vi "Facade.vi"(0 "Data In":T4, 2 "Display State In":T2, 3 "Container State":T3) -> (6 "Data Out":T4, 7 "Display State Out":T2, 8 "Action":T1)   [LabVIEW 2015, in "SAM.xctl"]
uses:
  SAM.xctl
  Data.vi
  Classes/Modulations/SAM/SAM.lvclass
  <vilib>/_xctls/Container State.ctl
  State.vi
  <vilib>/_xctls/Action.ctl
  Classes/Modulations/SAM/SAM.lvclass/SAM.ctl
  Classes/Modulations/SAM/Read Frequency (Hz).vi
  Classes/Modulations/SAM/Read Phase (0-1).vi
  Classes/Modulations/SAM/Write Frequency (Hz).vi
  Classes/Modulations/SAM/Write Phase (0-1).vi
  <vilib>/_xctls/XControlSupport.lvlib
panel:
  in  "Phase (cycles)":dbl min=0.0 max=1.0
  in  "Frequency (Hz)":dbl
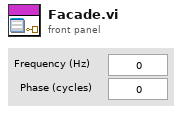
[diagram p1: front panel]
types:
  T1 = typedef "XControlSupport.lvlib/Action.ctl" = cluster{"Data Changed?":bool, "State Changed?":bool, "Action Name":string}
  T2 = typedef "SAM.xctl/State.vi" = cluster{"Numeric":dbl}
  T3 = typedef "XControlSupport.lvlib/Container State.ctl" = cluster{"Indicator?":bool, "Run Mode?":bool, " Refnum":refnum<vi>}
  T4 = typedef "SAM.xctl/Data.vi" = refnum<class "SAM.lvclass">
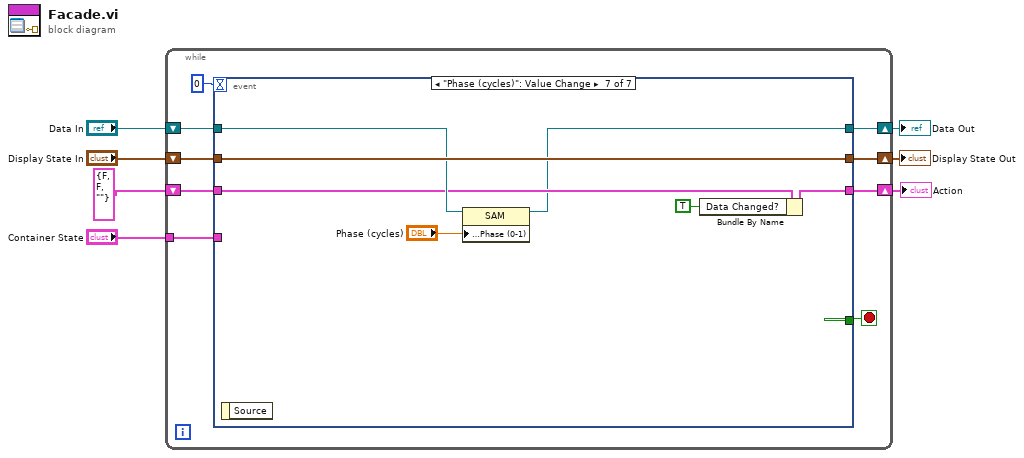
[diagram p0: block diagram]
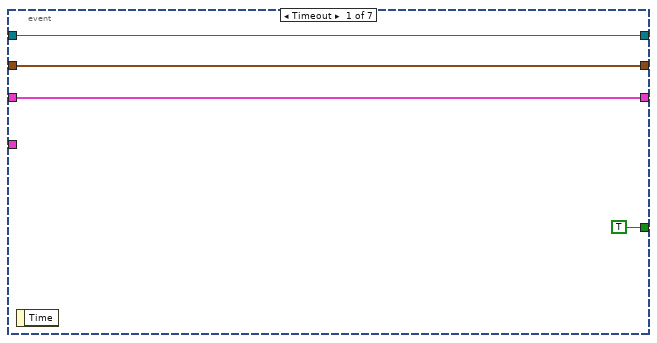
[diagram p2: hidden frame]
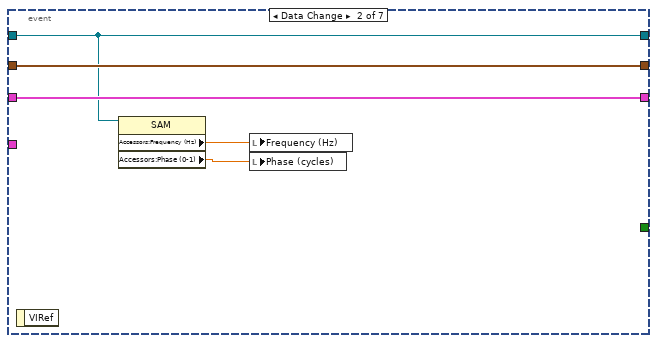
[diagram p3: hidden frame]
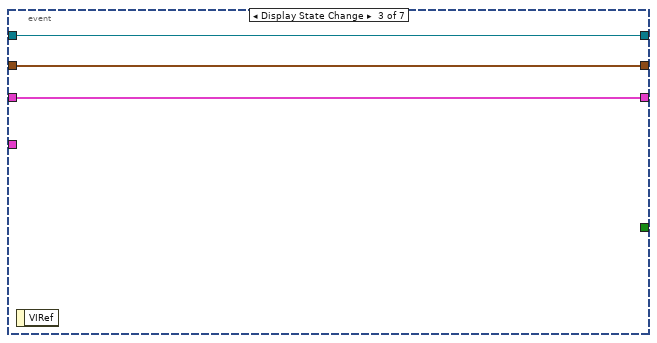
[diagram p4: hidden frame]
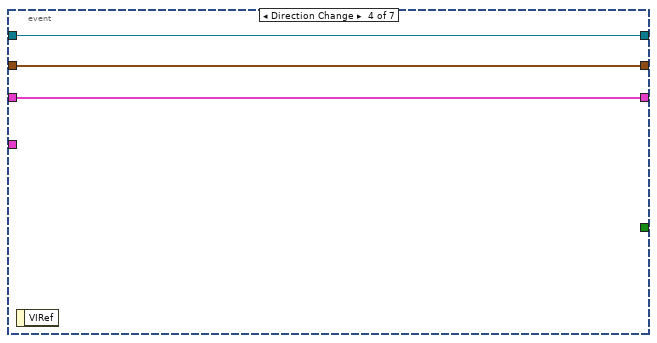
[diagram p5: hidden frame]
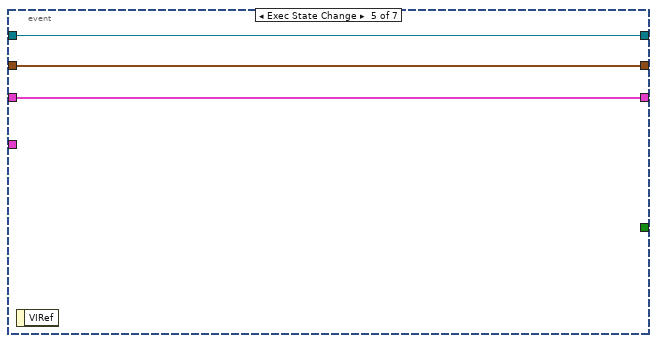
[diagram p6: hidden frame]
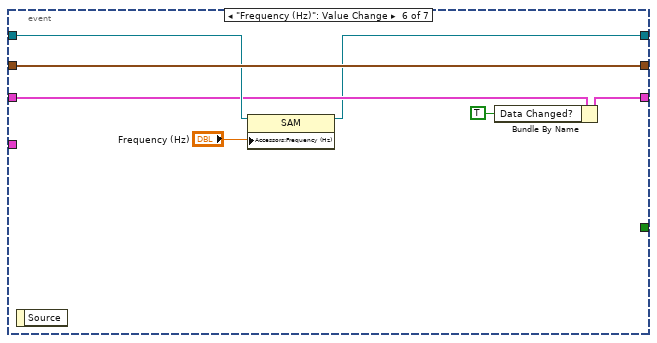
[diagram p7: hidden frame]
diagram:
  n1 = while {
    shift-right: [w15] -> w4
    shift-left: "Display State In" -> [w16]
    tunnel: "Container State" -> [w12]
    shift-right: [w10] -> w7
    shift-left: "Data In" -> [w11]
    shift-right: [w8] -> w2
    shift-left: T1 {"Data Changed?"=FALSE, "State Changed?"=FALSE, "Action Name"=""} ("Action") -> [w9]
    stop <- w14 stop-if-true
    n2 = event shown="[6] \"Phase (cycles)\": Value Change" {
      selector: _ -> [_ _ _ _ _ _ _]
      dyn-events: _ -> [_ _ _ _ _ _ _]
      timeout: 0 -> [_ _ _ _ _ _ _]
      tunnel: w16 -> [w18 w25 w28 w31 w34 w41 w48]
      tunnel: [w18 w25 w28 w31 w34 w41 w48] -> w15
      tunnel: [TRUE _ _ _ _ _ _] -> w14
      tunnel: w12 -> [_ _ _ _ _ _ _]
      tunnel: w11 -> [w17 w23 w27 w30 w33 w40 w47]
      tunnel: [w17 w23 w27 w30 w33 w38 w45] -> w10
      tunnel: [w19 w24 w26 w29 w32 w37 w44] -> w8
      tunnel: w9 -> [w19 w24 w26 w29 w32 w39 w46]
      event Timeout {
        n3 = event-data() -> ()  [unwired: 1 in, 1 out]
      }
      event Data Change {
        n4 = event-data() -> ()  [unwired: 1 in, 1 out]
        n5 = property class="SAM"(reference=w23) -> ("Accessors:Frequency (Hz)"=w22:dbl, "Accessors:Phase (0-1)"=w21:dbl)  [unwired: 1 in, 2 out]
        n6 = local write "Frequency (Hz)"(w22) -> ()
        n7 = local write "Phase (cycles)"(w21) -> ()
      }
      event Display State Change {
        n8 = event-data() -> ()  [unwired: 1 in, 1 out]
      }
      event Direction Change {
        n9 = event-data() -> ()  [unwired: 1 in, 1 out]
      }
      event Exec State Change {
        n10 = event-data() -> ()  [unwired: 1 in, 1 out]
      }
      event "Frequency (Hz)": Value Change {
        n11 = event-data() -> ()  [unwired: 1 in, 1 out]
        n12 = property class="SAM"(reference=w40, "Accessors:Frequency (Hz)"="Frequency (Hz)") -> (reference out=w38:T4)  [unwired: 1 in, 1 out]
        n13 = Bundle By Name(cluster=w39, "Data Changed?"=TRUE) -> (w37:T1)
      }
      event "Phase (cycles)": Value Change {
        n14 = event-data() -> ()  [unwired: 1 in, 1 out]
        n15 = property class="SAM"(reference=w47, "Accessors:Phase (0-1)"="Phase (cycles)") -> (reference out=w45:T4)  [unwired: 1 in, 1 out]
        n16 = Bundle By Name(cluster=w46, "Data Changed?"=TRUE) -> (w44:T1)
      }
    }
  }
  "Display State Out" <- w4
  "Data Out" <- w7
  "Action" <- w2
